vi "Save_Data_From_Analisis.vi"(8 "error in (no error)":errorcluster, 11 "Data":T1) -> (0 "error out":errorcluster)   [LabVIEW 2019, in "Save DB_SQLite.lvlib"]
doc: "All the analized data is saved in a DB of SQLite \n_____\nCreated using Delacor QMH Event Scripter 5.0.0.112."
uses:
  Save DB_SQLite.lvlib
  Save_Data_From_Analisis Argument--cluster.ctl
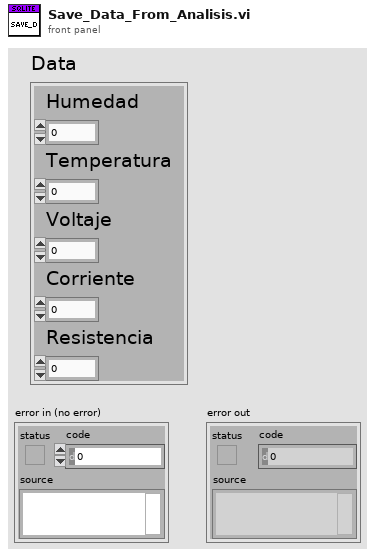
[diagram p1: front panel]
types:
  T1 = cluster{"Humedad":dbl, "Temperatura":dbl, "Voltaje":dbl, "Corriente":dbl, "Resistencia":i32}
  T2 = typedef "Save DB_SQLite.lvlib/Save_Data_From_Analisis Argument--cluster.ctl" = cluster{"Data":cluster{"Humedad":dbl, "Temperatura":dbl, "Voltaje":dbl, "Corriente":dbl, "Resistencia":i32}}
  T3 = typedef "Save DB_SQLite.lvlib/Request Events--cluster.ctl" = cluster{"Stop Module":refnum<user-event>, "Show Panel":refnum<user-event>, "Hide Panel":refnum<user-event>, "Get Module Execution Status":refnum<user-event>, "Show Diagram":refnum<user-event>, "Start Helper Loop":refnum<user-event>, "Stop helper loop":refnum<user-event>, "Set Waveform":refnum<user-event>, "Save_Data_From_Analisis":refnum<user-event>}
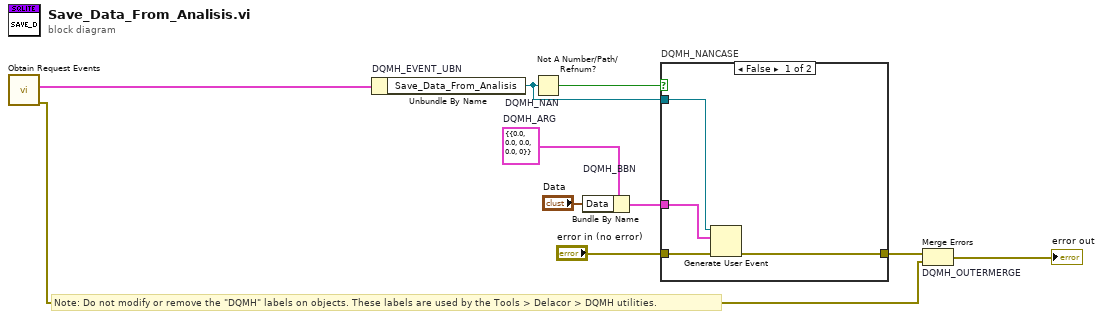
[diagram p0: block diagram]
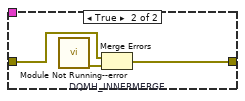
[diagram p2: hidden frame]
diagram:
  w2 = T2 {"Data"={"Humedad"=0.0, "Temperatura"=0.0, "Voltaje"=0.0, "Corriente"=0.0, "Resistencia"=0}}  # DQMH_ARG
  # "Note: Do not modify or remove the \"DQMH\" labels on objects. These labels are used by the Tools > Delacor > DQMH utilities."
  n1 = call "Obtain Request Events.vi"() -> ("error out"=w4:errorcluster, "Save DB_SQLite Request Events"=w3:T3)  [unwired: 10 in]
  n2 = Unbundle By Name "DQMH_EVENT_UBN"(w3) -> ("Save_Data_From_Analisis"=w6:refnum<user-event>)
  n3 = Not A Number/Path/Refnum? "DQMH_NAN"(number/path/refnum=w6) -> (NaN/Path/Refnum?=w7:bool)
  n4 = Bundle By Name "DQMH_BBN"(cluster=w2, "Data"="Data") -> (w8:T2)
  n5 = case "DQMH_NANCASE" shown="False" w7 {
    tunnel: "error in (no error)" -> [w14 w17]
    tunnel: [w13 w16] -> w5
    tunnel: w6 -> [w12 _]
    tunnel: w8 -> [w11 _]
    frame False {
      n6 = Generate User Event(user event=w12, event data cluster=w11, error in=w14) -> (error out=w13:errorcluster)  [unwired: 1 in, 1 out]
    }
    frame True {
      n7 = call "Module Not Running--error.vi"() -> ("error out"=w15:errorcluster)  [unwired: 11 in]
      n8 = Merge Errors "DQMH_INNERMERGE"(w17, w15) -> (w16:errorcluster)
    }
  }
  n9 = Merge Errors "DQMH_OUTERMERGE"(w5, w4) -> (→"error out":errorcluster)
